vi "Do.vi"(8 "error in (no error)":errorcluster, 10 "Actor in":refnum<class "Actor.lvclass">, 11 "Conceret Test Channel Move In Next Msg in":refnum<class "Conceret Test Channel Move In Next Msg.lvclass">) -> (0 "error out":errorcluster, 2 "Actor out":refnum<class "Actor.lvclass">)   [LabVIEW 2013, in "Test Channel View.lvlib" / "Conceret Test Channel Move In Next Msg.lvclass"]
doc: "(<B>Filename</B>: Actor Framework.lvlib:Message.lvclass:Do.vi)\n\nDefines what a message does when it is received by an actor. Generally, a message instructs an actor to invoke one of its methods.\n\nBy default, this method does nothing. A child class must override it to define behavior. Create a child class by using the Actor Framework Message Maker dialog box."
uses:
  Conceret Test Channel Move In Next Msg.lvclass
  <vilib>/ActorFramework/Actor/Actor.lvclass
  Test Channel View/Test Channel View.lvclass
  Models/Test Channel Model Messages/Abstract Test Channel Move In Next Msg/Abstract Test Channel Move In Next Msg.lvclass
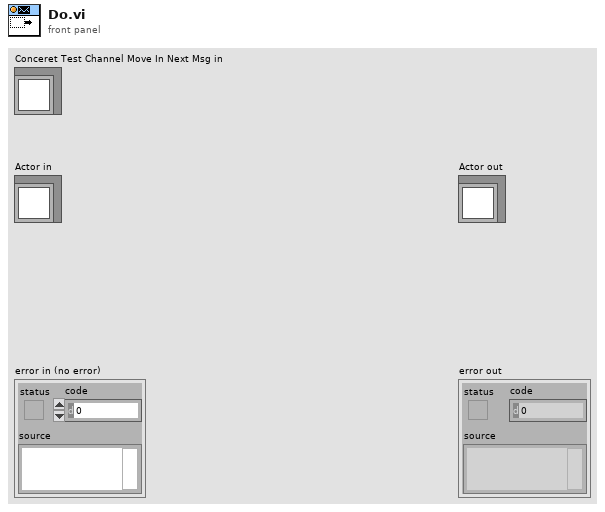
[diagram p1: front panel]
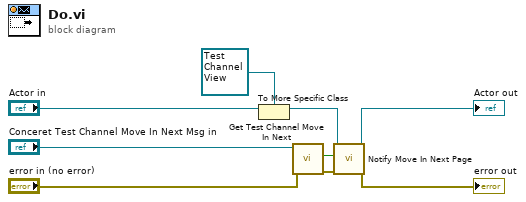
[diagram p0: block diagram]
diagram:
  n1 = To More Specific Class(target class=refnum<class "Test Channel View.lvclass"> refnum ("Test Channel View.lvlib:Test Channel View.lvclass"), reference="Actor in") -> (specific class reference=w6:refnum<class "Test Channel View.lvclass">)  [unwired: 1 in, 1 out]
  n2 = call "Get Test Channel Move In Next.vi"("error in (no error)"="error in (no error)", "Abstract Test Channel Move In Next Msg in"="Conceret Test Channel Move In Next Msg in") -> ("error out"=w5:errorcluster, "Test Channel Move In Next"=w1:bool)  [unwired: 7 in, 1 out]
  n3 = call "Notify Move In Next Page.vi"("error in (no error)"=w5, "Test Channel Move In Next"=w1, "Test Channel View in"=w6) -> ("error out"=→"error out":errorcluster, "Test Channel View out"=→"Actor out":refnum<class "Test Channel View.lvclass">)  [unwired: 7 in]
